vi "MUX Global.vi"() -> ()   [LabVIEW 2013, in "MUX Custom Device.lvlib"]
uses:
  MUX Custom Device.lvlib
panel:
  in  "Main Prop Names":string[](array[string])=["Physical Address", "Topology Name"]
  in  "Relay Prop. Names":string[](array[string])=["Relay Name"]
  in  "Dig Out":string="Digital Output"
  in  "Relay Ch GUID":string="b7606957-8ed9-4652-a85b-1af88f81eb0e"
  in  "Relay Ch":string="Relay Channel"
  in  "Sub Relay GUID":string="f32baacb-0ae2-4499-b68e-b9a8bc9bfad0"
  in  "Sub Relay":string="Relays"
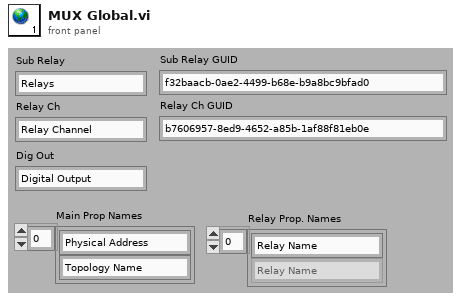
[diagram p1: front panel]
diagram:
